vi "readDataIn.vi"(8 "error in (no error)":errorcluster) -> (0 "error out":errorcluster, 3 "JSON string":string)   [LabVIEW 2017]
uses:
  TypeDefs/dataFGVState.ctl
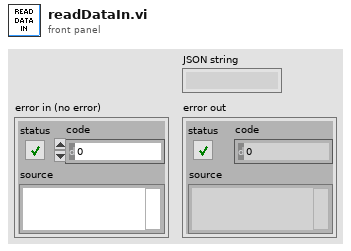
[diagram p1: front panel]
types:
  T1 = typedef "dataFGVState.ctl" = enum16{"init", "write data out", "read data out", "write data in", "read data in"}
  T2 = typedef "dataIn.ctl" = cluster{"Xtarget":dbl, "Ytarget":dbl, "Ztarget":dbl, "X_Attractor1":dbl, "Y_Attractor1":dbl, "Z_Attractor1":dbl, "X_Attractor2":dbl, "Y_Attractor2":dbl, "Z_Attractor2":dbl, "Traj_Flag":bool, "DeadZone":dbl, "Assistance":bool, "Shutdown":bool, "AssistanceLevel":dbl}
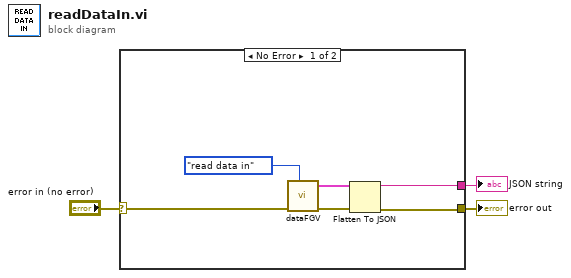
[diagram p0: block diagram]
diagram:
  n1 = case shown="No Error" "error in (no error)" {
    selector: "error in (no error)" -> [w8 w10]
    tunnel: [w5 w10] -> w2
    tunnel: [w4 _] -> w1
    frame No Error {
      n2 = call "dataFGV.vi"("Enum"=dataFGVState."read data in", "error in (no error)"=w8) -> ("error out"=w6:errorcluster, "DataIn"=w7:T2)  [unwired: 7 in, 1 out]
      n3 = Flatten To JSON(anything=w7, error in (no error)=w6) -> (JSON string=w4:string, 11:w5:errorcluster)  [unwired: 1 in]
    }
    frame Error {
    }
  }
  "error out" <- w2
  "JSON string" <- w1
